vi "Reset.vi"(8 "error in (no error)":errorcluster, 10 "Message in":refnum<class "ResetMessage.lvclass">, 11 "Thorcam in":refnum<class "Thorcam.lvclass">) -> (0 "error out":errorcluster, 3 "Thorcam out":refnum<class "Thorcam.lvclass">)   [LabVIEW 2012, in "Thorcam.lvclass"]
doc: "The reset method processes the command 'reset'. \n\nResets the internal state of the component (without performing a full initialisation). This could be resetting hardware, or private data to default values."
uses:
  Thorcam.lvclass
  <vilib>/Distrio/Murmex/ResetMessage/ResetMessage.lvclass
  <vilib>/Distrio/Murmex/Murmex/Murmex.lvclass
  Thorcam.lvclass/Thorcam.ctl
panel:
  # "This method is called when the RESET\ntrigger is sent. \n\nOverride this method when your component needs to\nrespond to this trigger. \n\nCall parent for proper implementation"
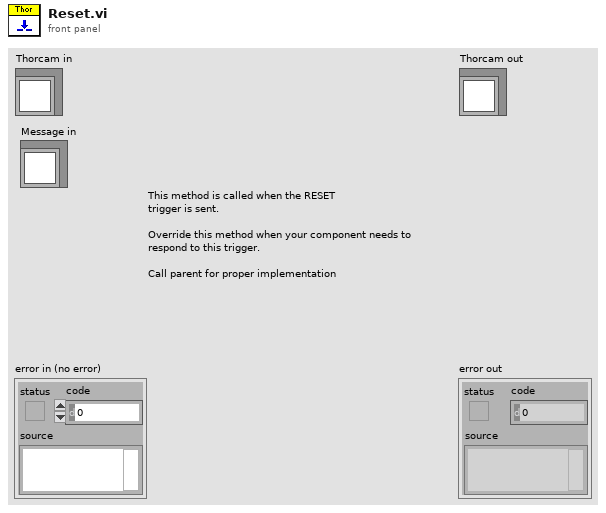
[diagram p1: front panel]
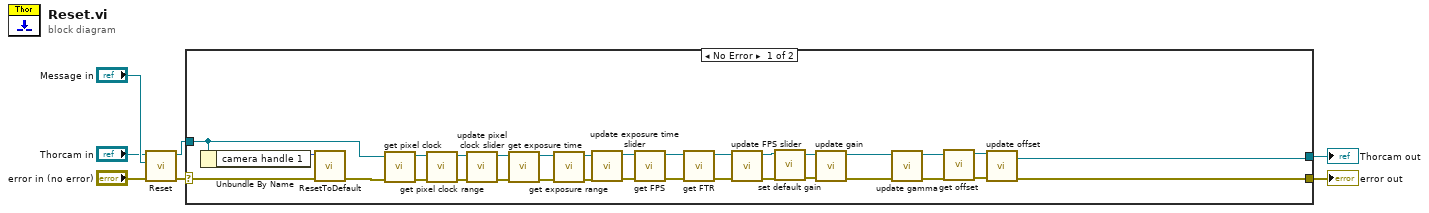
[diagram p0: block diagram]
diagram:
  n1 = call-parent "Reset.vi"("error in (no error)"="error in (no error)", "Message in"="Message in", "Murmex in"="Thorcam in") -> ("error out"=w4:errorcluster, "Murmex out"=w2:refnum<class "Thorcam.lvclass">)  [unwired: 7 in]
  n2 = case shown="No Error" w4 {
    selector: w4 -> [w39 w41]
    tunnel: [w34 w41] -> w3
    tunnel: w2 -> [w36 w40]
    tunnel: [w35 w40] -> w1
    frame No Error {
      n3 = Unbundle By Name(w36) -> ("camera handle 1"=w38:u32)
      n4 = call <instrlib>:"ResetToDefault.vi"("error in"=w39, "Camera Handle In"=w38) -> ("error out"=w37:errorcluster)  [unwired: 8 in, 1 out]
      n5 = call-dynamic "get pixel clock.vi"("error in (no error)"=w37, "Thorcam in"=w36) -> ("error out"=w32:errorcluster, "Thorcam out"=w33:refnum<class "Thorcam.lvclass">)  [unwired: 8 in]
      n6 = call-dynamic "get pixel clock range.vi"("error in (no error)"=w32, "Thorcam in"=w33) -> ("error out"=w31:errorcluster, "Thorcam out"=w30:refnum<class "Thorcam.lvclass">)  [unwired: 8 in]
      n7 = call-dynamic "update pixel clock slider.vi"("error in (no error)"=w31, "Thorcam in"=w30) -> ("error out"=w28:errorcluster, "Thorcam out"=w29:refnum<class "Thorcam.lvclass">)  [unwired: 8 in]
      n8 = call-dynamic "get exposure time.vi"("error in (no error)"=w28, "Thorcam in"=w29) -> ("error out"=w26:errorcluster, "Thorcam out"=w27:refnum<class "Thorcam.lvclass">)  [unwired: 7 in, 1 out]
      n9 = call-dynamic "get exposure range.vi"("error in (no error)"=w26, "Thorcam in"=w27) -> ("error out"=w24:errorcluster, "Thorcam out"=w25:refnum<class "Thorcam.lvclass">)  [unwired: 8 in]
      n10 = call-dynamic "update exposure time slider.vi"("error in (no error)"=w24, "Thorcam in"=w25) -> ("error out"=w22:errorcluster, "Thorcam out"=w23:refnum<class "Thorcam.lvclass">)  [unwired: 8 in]
      n11 = call-dynamic "get FPS.vi"("error in (no error)"=w22, "Thorcam in"=w23) -> ("error out"=w20:errorcluster, "Thorcam out"=w21:refnum<class "Thorcam.lvclass">)  [unwired: 8 in]
      n12 = call-dynamic "get FTR.vi"("error in (no error)"=w20, "Thorcam in"=w21) -> ("error out"=w18:errorcluster, "Thorcam out"=w19:refnum<class "Thorcam.lvclass">)  [unwired: 8 in]
      n13 = call-dynamic "update FPS slider.vi"("error in (no error)"=w18, "Thorcam in"=w19) -> ("error out"=w9:errorcluster, "Thorcam out"=w11:refnum<class "Thorcam.lvclass">)  [unwired: 8 in]
      n14 = call-dynamic "set default gain.vi"("error in (no error)"=w9, "Thorcam in"=w11) -> ("error out"=w8:errorcluster, "Thorcam out"=w10:refnum<class "Thorcam.lvclass">)  [unwired: 8 in]
      n15 = call-dynamic "update gain.vi"("error in (no error)"=w8, "Thorcam in"=w10) -> ("error out"=w12:errorcluster, "Thorcam out"=w13:refnum<class "Thorcam.lvclass">)  [unwired: 8 in]
      n16 = call-dynamic "update gamma.vi"("error in (no error)"=w12, "Thorcam in"=w13) -> ("error out"=w14:errorcluster, "Thorcam out"=w15:refnum<class "Thorcam.lvclass">)  [unwired: 8 in]
      n17 = call-dynamic "get offset.vi"("error in (no error)"=w14, "Thorcam in"=w15) -> ("error out"=w16:errorcluster, "Thorcam out"=w17:refnum<class "Thorcam.lvclass">)  [unwired: 8 in]
      n18 = call-dynamic "update offset.vi"("error in (no error)"=w16, "Thorcam in"=w17) -> ("error out"=w34:errorcluster, "Thorcam out"=w35:refnum<class "Thorcam.lvclass">)  [unwired: 8 in]
    }
    frame Error {
    }
  }
  "error out" <- w3
  "Thorcam out" <- w1
